vi "Generate Survey Waypoints.vi"(5 "Camera Settings":T2, 7 "Altitude (m)":dbl, 9 "Overlap (%)":dbl, 11 "error in (no error)":errorcluster) -> (4 "Grid Waypoints":T1[](array[typedef]) {"Latitude" format="%#_10g"; "Longitude" format="%#_10g"}, 6 "Frame Height (m)":dbl, 15 "error out":errorcluster)   [LabVIEW 2014]
uses:
  Settings File/Controls/Camera Settings.ctl
  Lat Long Conversion/Controls/PointLatLon.ctl
  Controls/Grid Waypoint States.ctl
  <vilib>/Analysis/NI_AAL_Geometry.lvlib
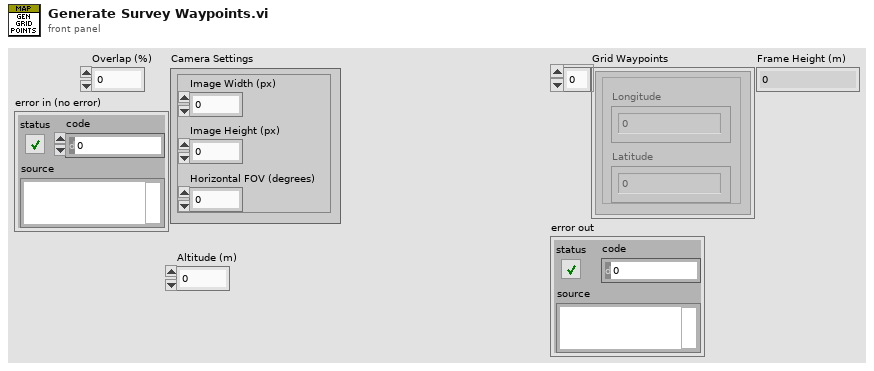
[diagram p1: front panel]
types:
  T1 = typedef "PointLatLon.ctl" = cluster{"Longitude":dbl, "Latitude":dbl}
  T2 = typedef "Camera Settings.ctl" = cluster{"Image Width (px)":dbl, "Image Height (px)":dbl, "Horizontal FOV (degrees)":dbl}
  T3 = typedef "Grid Waypoint States.ctl" = enum16{"Is Point in Polygon?", "Does Frame Intersect Polygon?", "Is Max LON Exceeded?", "Is Max/Min Lat Exceeded?", "Increment Lat", "Increment Lon", "Add Waypoint"}
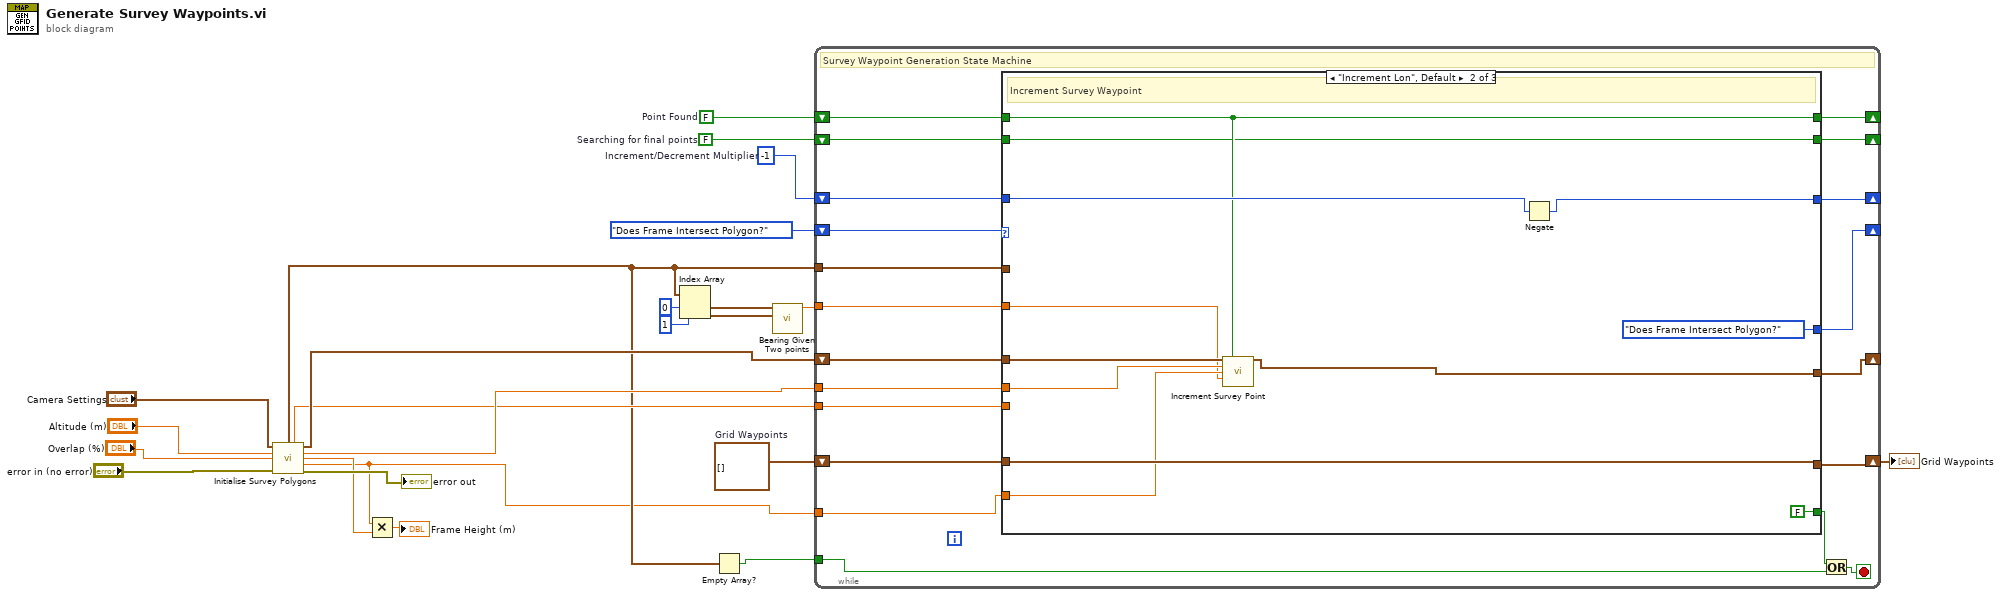
[diagram p0: block diagram]
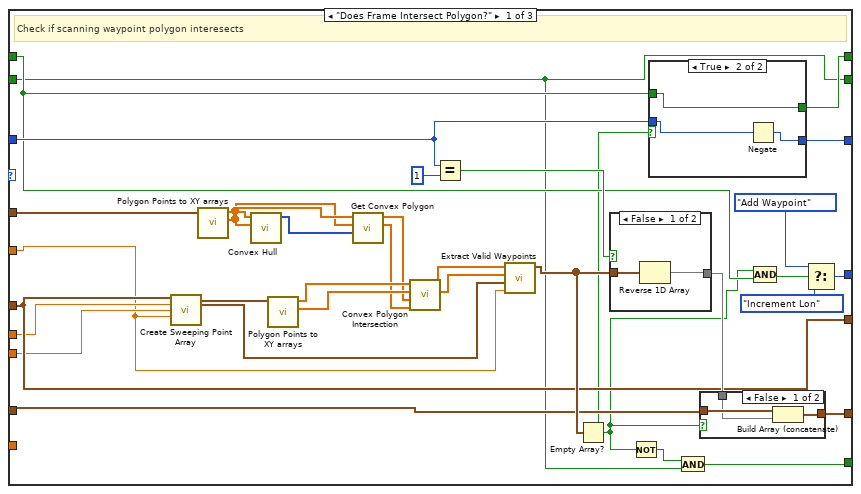
[diagram p2: hidden frame]
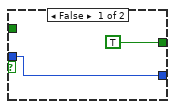
[diagram p3: hidden frame]
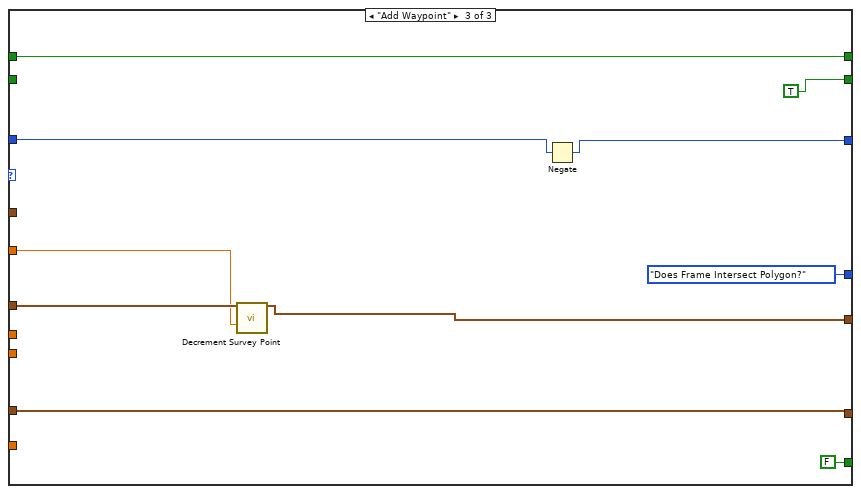
[diagram p6: hidden frame]
diagram:
  w4 = FALSE  # Searching for final points
  w9 = FALSE  # Point Found
  w23 = -1  # Increment/Decrement Multiplier
  w5 = T1[] []  # Grid Waypoints
  n1 = call "Initialise Survey Polygons.vi"("Camera Settings"="Camera Settings", "Altitude (m)"="Altitude (m)", "Overlap (%)"="Overlap (%)", "Error In"="error in (no error)") -> ("Points of Polygon"=w12:T1[], "Diameter (km)"=w14:dbl, "Start Point"=w16:T1, "Image Width (m)"=w15:dbl, "Image Height (m)"=w3:dbl, "Overlap Adjustment (0-1)"=w2:dbl, "Error Out"=→"error out":errorcluster)  [unwired: 5 in]
  n2 = Multiply(x=w2, y=w3) -> (x*y=→"Frame Height (m)":dbl)
  n3 = Index Array(array=w12, index #1=0 ("index"), index #2=1 ("index")) -> (element #1=w8:T1, element #2=w7:T1)
  n4 = Empty Array?(array=w12) -> (empty?=w6:bool)
  n5 = call "Bearing Given Two points.vi"("End Point"=w7, "Origin Point"=w8) -> ("Bearing (True North)"=w10:dbl)  [unwired: 8 in, 1 out]
  n6 = while {
    shift-right: [w41] -> _
    shift-left: Grid_Waypoint_States."Does Frame Intersect Polygon?" ("Grid Waypoint State") -> [w44]
    shift-right: [w38] -> _
    shift-left: w16 -> [w43]
    shift-right: [w35] -> w22
    shift-left: w5 -> [w31]
    tunnel: w12 -> [w42]
    tunnel: w15 -> [w40]
    shift-right: [w36] -> _
    shift-left: w23 -> [w39]
    tunnel: w2 -> [w37]
    tunnel: w6 -> [w32]
    tunnel: w14 -> [w30]
    tunnel: w10 -> [w29]
    shift-right: [w27] -> _
    shift-left: w9 -> [w28]
    shift-right: [w25] -> _
    shift-left: w4 -> [w26]
    stop <- w33 stop-if-true
    # "Survey Waypoint Generation State Machine"
    n7 = case shown="\"Increment Lon\", Default" w44 {
      tunnel: w43 -> [w62 w97 w107]
      tunnel: w31 -> [w55 w100 w110]
      tunnel: w42 -> [w61 _ _]
      tunnel: [w52 Grid_Waypoint_States."Does Frame Intersect Polygon?" ("f") Grid_Waypoint_States."Does Frame Intersect Polygon?" ("f")] -> w41
      tunnel: w40 -> [w60 w96 _]
      tunnel: [w45 FALSE FALSE] -> w34
      tunnel: w39 -> [w70 w99 w109]
      tunnel: [w62 w93 w105] -> w38
      tunnel: w37 -> [_ w95 _]
      tunnel: [w69 w98 w108] -> w36
      tunnel: [w76 w100 w110] -> w35
      tunnel: w30 -> [w59 _ _]
      tunnel: w29 -> [w57 w94 w106]
      tunnel: w28 -> [w53 w92 w104]
      tunnel: [w54 w92 w104] -> w27
      tunnel: w26 -> [w48 w91 _]
      tunnel: [w48 w91 TRUE] -> w25
      frame "Does Frame Intersect Polygon?" {
        # "Check if scanning waypoint polygon interesects"
        n8 = call "Create Sweeping Point Array.vi"("Origin Point"=w62, "Image Width (m)"=w60, "Diameter of polygon (km)"=w59, "Bearing of first two points"=w57) -> ("Frame Points"=w56:T1[], "Bottom RIght corner"=w58:T1)  [unwired: 9 in, 1 out]
        n9 = call "Polygon Points to XY arrays.vi"("Polygon Points"=w61) -> ("Y Array"=w66:dbl[], "X Array"=w67:dbl[])  [unwired: 9 in]
        n10 = call <vilib>:"Convex Hull.vi"("Y"=w66, "X"=w67) -> ("Convex Hull"=w65:i32[])  [unwired: 8 in, 1 out]
        n11 = call "Polygon Points to XY arrays.vi"("Polygon Points"=w56) -> ("Y Array"=w73:dbl[], "X Array"=w72:dbl[])  [unwired: 9 in]
        n12 = call "Get Convex Polygon.vi"("Convex Hull Points"=w65, "y"=w66, "X"=w67) -> ("Y"=w64:dbl[], "X"=w63:dbl[])  [unwired: 7 in]
        n13 = call <vilib>:"Convex Polygon Intersection.vi"("Y 2"=w64, "X 2"=w63, "Y 1"=w73, "X 1"=w72) -> ("Intersection Y"=w77:dbl[], "Intersection X"=w78:dbl[])  [unwired: 5 in, 1 out]
        n14 = Equal?(x=w70, y=1) -> (x = y?=w75:bool)
        n15 = call "Extract Valid Waypoints.vi"("Bearing"=w57, "Origin Point"=w58, "Y intersects"=w77, "X Intersects"=w78) -> ("Valid Points"=w71:T1[])  [unwired: 7 in]
        n16 = Empty Array?(array=w71) -> (empty?=w47:bool)
        n17 = case shown="False" w75 {
          tunnel: [w88 w90] -> w74
          tunnel: w71 -> [w89 w90]
          frame False {
            n18 = Reverse 1D Array(array=w89) -> (reversed array=w88:T1[])
          }
          frame True {
          }
        }
        n19 = Not(x=w47) -> (.not. x?=w46:bool)
        n20 = case shown="True" w47 {
          tunnel: w70 -> [w80 w83]
          tunnel: [w80 w82] -> w69
          tunnel: w53 -> [_ w81]
          tunnel: [TRUE w81] -> w54
          frame False {
          }
          frame True {
            n21 = Negate(x=w83) -> (-x=w82:i32)
          }
        }
        n22 = And(x=w46, y=w48) -> (x .and. y?=w45:bool)
        n23 = case shown="False" w47 {
          tunnel: w55 -> [w86 w87]
          tunnel: [w85 w87] -> w76
          tunnel: w74 -> [w84 _]
          frame False {
            n24 = Build Array (concatenate)(w86, w84) -> (w85:T1[])
          }
          frame True {
          }
        }
        n25 = Compound Arithmetic op=AND(w47, w53) -> (w50:bool)
        n26 = Select(t=Grid_Waypoint_States."Add Waypoint" ("f"), s=w50, f=Grid_Waypoint_States."Increment Lon") -> (s? t:f=w52:T3)
      }
      frame "Increment Lon", Default {
        # "Increment Survey Waypoint"
        n27 = call "Increment Survey Point.vi"("Current Point"=w97, "Point Found"=w92, "Image Width (m)"=w96, "Overlap Adjustment"=w95, "Bearing"=w94) -> ("New Point"=w93:T1)  [unwired: 9 in, 1 out]
        n28 = Negate(x=w99) -> (-x=w98:i32)
      }
      frame "Add Waypoint" {
        n29 = call "Decrement Survey Point.vi"("Current Point"=w107, "Bearing"=w106) -> ("New Point"=w105:T1)  [unwired: 12 in, 1 out]
        n30 = Negate(x=w109) -> (-x=w108:i32)
      }
    }
    n31 = Or(x=w34, y=w32) -> (x .or. y?=w33:bool)
  }
  "Grid Waypoints" <- w22
